vi "Write PID Parameters.vi"(8 "error in (no error)":errorcluster, 10 "PID Parameters":T1, 11 "PID Loop in":refnum<class "PID Loop.lvclass">) -> (0 "error out":errorcluster, 3 "PID Loop out":refnum<class "PID Loop.lvclass">)   [LabVIEW 2014, in "PID Loop.lvclass"]
uses:
  PID Loop.lvclass
  PID Parameters.ctl
  PID Loop.lvclass/PID Loop.ctl
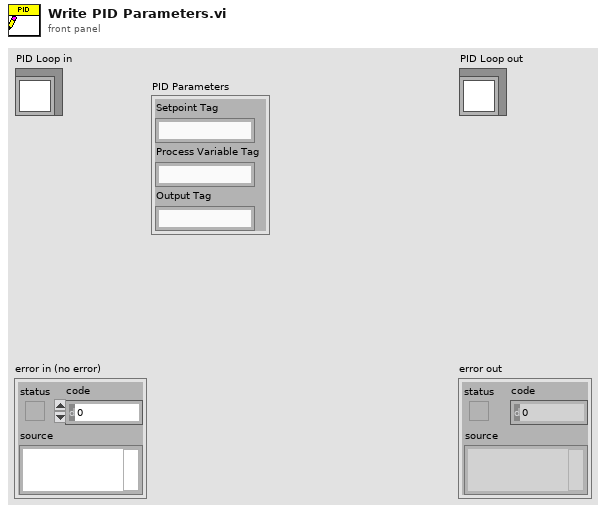
[diagram p1: front panel]
types:
  T1 = typedef "PID Loop.lvclass/PID Parameters.ctl" = cluster{"Setpoint Tag":string, "Process Variable Tag":string, "Output Tag":string}
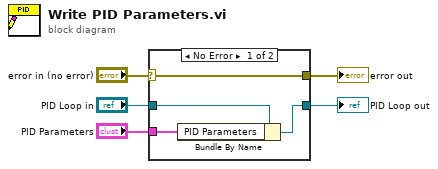
[diagram p0: block diagram]
diagram:
  n1 = case shown="No Error" "error in (no error)" {
    selector: "error in (no error)" -> [w9 w10]
    tunnel: [w9 w10] -> w4
    tunnel: [w7 w11] -> w2
    tunnel: "PID Loop in" -> [w8 w11]
    tunnel: "PID Parameters" -> [w6 _]
    frame No Error {
      n2 = Bundle By Name(cluster=w8, "PID Parameters"=w6) -> (w7:refnum<class "PID Loop.lvclass">)
    }
    frame Error {
    }
  }
  "error out" <- w4
  "PID Loop out" <- w2
